vi "visionDisc.vi"(4 "Blue or Luma or Val or Inten Range (Color Threshold 1)":cluster{"Lower value":i32, "Upper value":i32}={"Lower value"=5, "Upper value"=250}, 5 "Green or Sat Range (Color Threshold 1)":cluster{"Lower value":i32, "Upper value":i32}={"Lower value"=43, "Upper value"=210}, 6 "Red or Hue Range (Color Threshold 1)":cluster{"Lower value":i32, "Upper value":i32}={"Lower value"=119, "Upper value"=255}, 7 "Image in":T1) -> (0 "error out":errorcluster, 1 "Particle Measurements (Pixels) (Particle Analysis 1)":dbl[][](array[numeric]) format="%.2f", 2 "Image Out":T1(plugin-control), 3 "Particle Measurements (Real-World) (Particle Analysis 1)":dbl[][](array[numeric]) format="%.2f")   [LabVIEW 2012]
uses:
  <vilib>/vision/Image Controls.llb/IMAQ Image.ctl
  <vilib>/vision/NI_Vision_Development_Module.lvlib
panel:
  out "Right Motor New":dbl
  out "Left Motor New":dbl
  in  "Right Motor":dbl
  in  "Left Motor":dbl
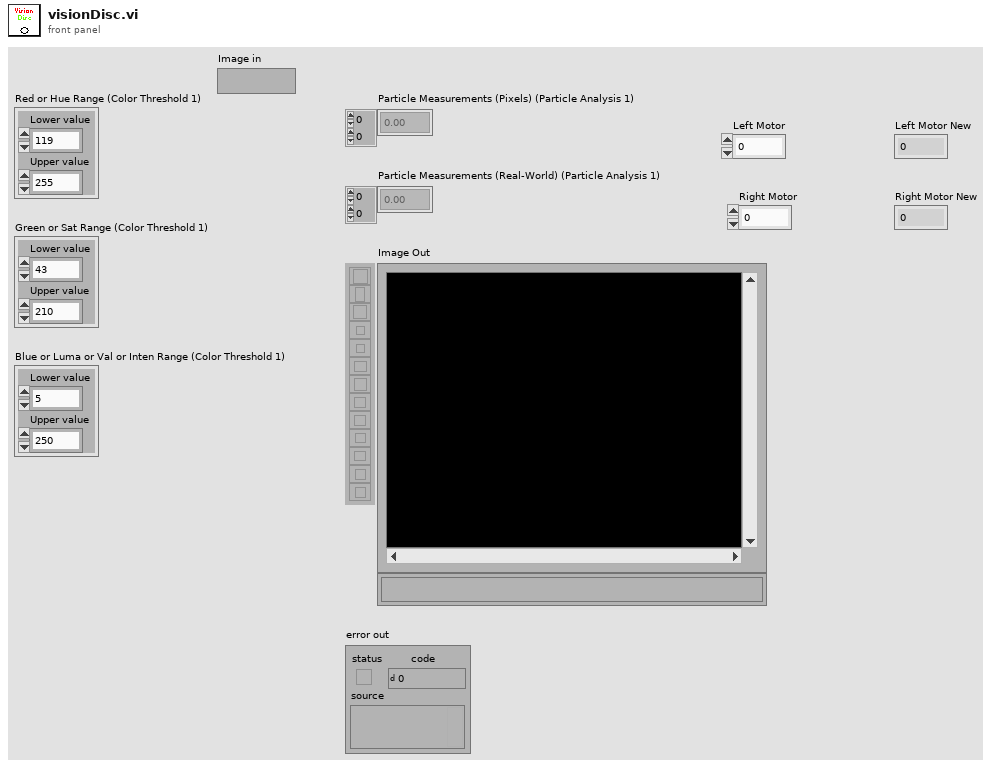
[diagram p1: front panel]
types:
  T1 = typedef "IMAQ Image.ctl" = refnum<image>
  T2 = typedef "Image Type" = u32
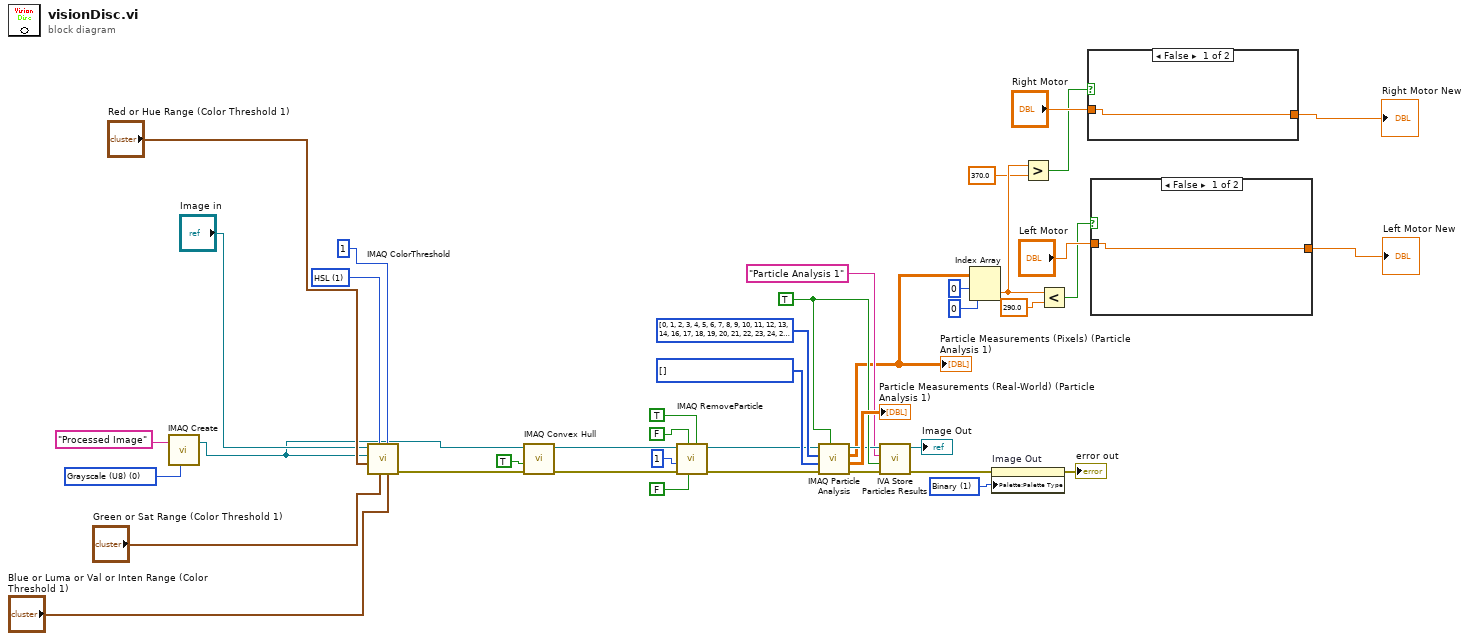
[diagram p0: block diagram]
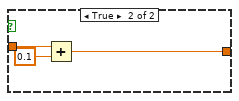
[diagram p2: hidden frame]
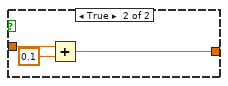
[diagram p3: hidden frame]
diagram:
  w4 = T2 0 items=["Grayscale (U8)", "Grayscale (I16)", "Grayscale (SGL)", "Complex (CSG)", "RGB (U32)", "HSL (U32)", "RGB (U64)"] ("Image Type")
  w20 = u32 1 items=["Grayscale", "Binary", "Gradient", "Rainbow", "Temperature", "User Defined"] ("Palette")
  w28 = i32[] [] items=["Center of Mass X", "Center of Mass Y", "First Pixel X", "First Pixel Y", "Bounding Rect Left", "Bounding Rect Top", "Bounding Rect Right", "Bounding Rect Bottom", "Max Feret Diameter Start X", "Max Feret Diameter Start Y", "Max Feret Diameter End X", "Max Feret Diameter End Y", "Max Horiz. Segment Length Left", "Max Horiz. Segment Length Right", "Max Horiz. Segment Length Row", "-", "Bounding Rect Width", "Bounding Rect Height", "Bounding Rect Diagonal", "Perimeter", "Convex Hull Perimeter", "Holes' Perimeter", "Max Feret Diameter", "Equivalent Ellipse Major Axis", "Equivalent Ellipse Minor Axis", "Equivalent Ellipse Minor Axis (Feret)", "Equivalent Rect Long Side", "Equivalent Rect Short Side", "Equivalent Rect Diagonal", "Equivalent Rect Short Side (Feret)", "Average Horiz. Segment Length", "Average Vert. Segment Length", "Hydraulic Radius", "Waddel Disk Diameter", "-", "Area", "Holes' Area", "Particle & Holes' Area", "Convex Hull Area", "Image Area", "-", "Number of Holes", "Number of Horiz. Segments", "Number of Vert. Segments", "-", "Orientation", "Max Feret Diameter Orientation", "-", "% Area/Image Area", "% Area/(Particle & Holes' Area)", "Ratio of Equivalent Ellipse Axes", "Ratio of Equivalent Rect Sides", "-", "Elongation Factor", "Compactness Factor", "Heywood Circularity Factor", "Type Factor", "-", "Sum X", "Sum Y", "Sum XX", "Sum XY", "Sum YY", "Sum XXX", "Sum XXY", "Sum XYY", "Sum YYY", "-", "Moment of Inertia XX", "Moment of Inertia XY", "Moment of Inertia YY", "Moment of Inertia XXX", "Moment of Inertia XXY", "Moment of Inertia XYY", "Moment of Inertia YYY", "Norm. Moment of Inertia XX", "Norm. Moment of Inertia XY", "Norm. Moment of Inertia YY", "Norm. Moment of Inertia XXX", "Norm. Moment of Inertia XXY", "Norm. Moment of Inertia XYY", "Norm. Moment of Inertia YYY", "Hu Moment 1", "Hu Moment 2", "Hu Moment 3", "Hu Moment 4", "Hu Moment 5", "Hu Moment 6", "Hu Moment 7"] ("Real-World Measurements")
  w29 = i32[] [0, 1, 2, 3, 4, 5, 6, 7, 8, 9, 10, 11, 12, 13, 14, 16, 17, 18, 19, 20, 21, 22, 23, 24, 25, 26, 27, 28, 29, 30, 31, 32, 33, 35, 36, 37, 38, 39, 41, 42, 43, 45, 46, 48, 49, 50, 51, 53, 54, 55, 56, 58, 59, 60, 61, 62, 63, 64, 65, 66, 68, 69, 70, 71, 72, 73, 74, 75, 76, 77, 78, 79, 80, 81, 82, 83, 84, 85, 86, 87, 88] items=["Center of Mass X", "Center of Mass Y", "First Pixel X", "First Pixel Y", "Bounding Rect Left", "Bounding Rect Top", "Bounding Rect Right", "Bounding Rect Bottom", "Max Feret Diameter Start X", "Max Feret Diameter Start Y", "Max Feret Diameter End X", "Max Feret Diameter End Y", "Max Horiz. Segment Length Left", "Max Horiz. Segment Length Right", "Max Horiz. Segment Length Row", "-", "Bounding Rect Width", "Bounding Rect Height", "Bounding Rect Diagonal", "Perimeter", "Convex Hull Perimeter", "Holes' Perimeter", "Max Feret Diameter", "Equivalent Ellipse Major Axis", "Equivalent Ellipse Minor Axis", "Equivalent Ellipse Minor Axis (Feret)", "Equivalent Rect Long Side", "Equivalent Rect Short Side", "Equivalent Rect Diagonal", "Equivalent Rect Short Side (Feret)", "Average Horiz. Segment Length", "Average Vert. Segment Length", "Hydraulic Radius", "Waddel Disk Diameter", "-", "Area", "Holes' Area", "Particle & Holes' Area", "Convex Hull Area", "Image Area", "-", "Number of Holes", "Number of Horiz. Segments", "Number of Vert. Segments", "-", "Orientation", "Max Feret Diameter Orientation", "-", "% Area/Image Area", "% Area/(Particle & Holes' Area)", "Ratio of Equivalent Ellipse Axes", "Ratio of Equivalent Rect Sides", "-", "Elongation Factor", "Compactness Factor", "Heywood Circularity Factor", "Type Factor", "-", "Sum X", "Sum Y", "Sum XX", "Sum XY", "Sum YY", "Sum XXX", "Sum XXY", "Sum XYY", "Sum YYY", "-", "Moment of Inertia XX", "Moment of Inertia XY", "Moment of Inertia YY", "Moment of Inertia XXX", "Moment of Inertia XXY", "Moment of Inertia XYY", "Moment of Inertia YYY", "Norm. Moment of Inertia XX", "Norm. Moment of Inertia XY", "Norm. Moment of Inertia YY", "Norm. Moment of Inertia XXX", "Norm. Moment of Inertia XXY", "Norm. Moment of Inertia XYY", "Norm. Moment of Inertia YYY", "Hu Moment 1", "Hu Moment 2", "Hu Moment 3", "Hu Moment 4", "Hu Moment 5", "Hu Moment 6", "Hu Moment 7"] ("Pixel Measurements")
  w24 = TRUE ("Connectivity 4/8 (8)")
  w41 = u16 1 items=["RGB", "HSL", "HSV", "HSI"] ("Color Mode")
  n1 = call "IMAQ Create"("Image Name"="Processed Image", "Image Type"=w4) -> ("New Image"=w2:T1)  [unwired: 2 in, 2 out]
  n2 = call "IMAQ ColorThreshold"("Blue or Luma or Val or Inten Range"="Blue or Luma or Val or Inten Range (Color Threshold 1)", "Replace Value"=1, "Green or Sat Range"="Green or Sat Range (Color Threshold 1)", "Color Mode"=w41, "Red or Hue Range"="Red or Hue Range (Color Threshold 1)", "Image Dst"=w2, "Image Src"="Image in") -> ("error out"=w37:errorcluster)  [unwired: 1 in, 3 out]
  n3 = call "IMAQ Convex Hull"("error in (no error)"=w37, "Connectivity 4/8 (8)"=TRUE, "Image Src"=w2) -> ("error out"=w30:errorcluster, "Image Dst Out"=w31:T1)  [unwired: 1 in, 6 out]
  n4 = call "IMAQ RemoveParticle"("Connectivity 4/8 (8)"=TRUE, "Low Pass/High Pass (Low)"=FALSE, "Square/Hexa (Square)"=FALSE, "error in (no error)"=w30, "Number of Erosion"=1, "Image Src"=w31) -> ("error out"=w26:errorcluster, "Image Dst Out"=w25:T1)  [unwired: 1 in, 3 out]
  n5 = call "IMAQ Particle Analysis"("Connectivity 4/8 (8)"=w24, "error in (no error)"=w26, "Real-World Measurements"=w28, "Pixel Measurements"=w29, "Image"=w25) -> ("error out"=w21:errorcluster, "Particle Measurements (Real-World)"=→"Particle Measurements (Real-World) (Particle Analysis 1)":dbl[][], "Particle Measurements (Pixels)"=w17:dbl[][], "Image Out (duplicate)"=w23:T1)  [unwired: 3 out]
  "Particle Measurements (Pixels) (Particle Analysis 1)" <- w17
  n6 = call <vilib>:"IVA Store Particles Results.vi"("error in (no error)"=w21, "Connectivity 4/8 (8)"=w24, "Step Name"="Particle Analysis 1", "Image in"=w23) -> ("error out"=w19:errorcluster, "Image dup"=→"Image Out":T1)  [unwired: 6 out]
  n7 = Index Array(array=w17, index (row)=0, index (col)=0 ("disabled index (col)")) -> (element=w11:dbl)
  n8 = property on="Image Out" class="ImageControl"(error in=w19, "Palette:Palette Type"=w20) -> (error out=→"error out":errorcluster)  [unwired: 1 in, 1 out]
  n9 = Greater?(x=w11, y=370.0) -> (0:w7:bool)
  n10 = Less?(x=w11, y=290.0) -> (x < y?=w6:bool)
  n11 = case shown="False" w7 {
    tunnel: "Right Motor" -> [w43 w46]
    tunnel: [w43 w45] -> w9
    frame False {
    }
    frame True {
      n12 = Add(x=w46, y=0.1) -> (x+y=w45:dbl)
    }
  }
  "Right Motor New" <- w9
  n13 = case shown="False" w6 {
    tunnel: "Left Motor" -> [w47 w50]
    tunnel: [w47 w49] -> w8
    frame False {
    }
    frame True {
      n14 = Add(x=w50, y=0.1) -> (x+y=w49:dbl)
    }
  }
  "Left Motor New" <- w8
